vi "read_data.vi"(8 "error in (no error)":errorcluster, 11 "SGDClassifier in":refnum<class "SGDClassifier.lvclass">) -> (0 "error out":errorcluster, 2 "data":T1, 3 "SGDClassifier out":refnum<class "SGDClassifier.lvclass">)   [LabVIEW 2020, in "SGDClassifier.lvclass"]
uses:
  SGDClassifier.lvclass
  Controls/sgdclassifier_data.ctl
  SGDClassifier.lvclass/SGDClassifier.ctl
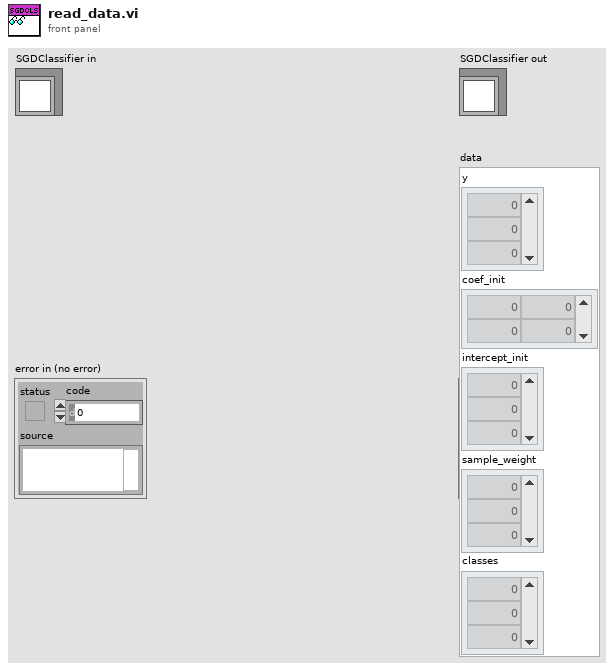
[diagram p1: front panel]
types:
  T1 = typedef "sgdclassifier_data.ctl" = cluster{"y":dbl[], "coef_init":dbl[][], "intercept_init":dbl[], "sample_weight":dbl[], "classes":dbl[]}
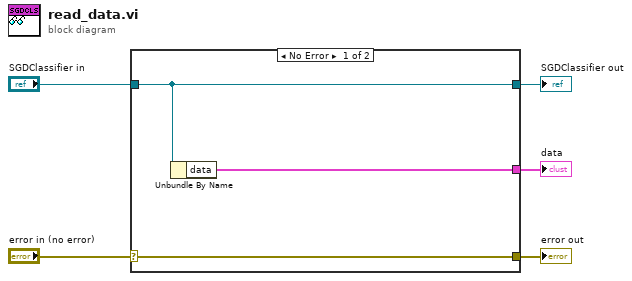
[diagram p0: block diagram]
diagram:
  n1 = case shown="No Error" "error in (no error)" {
    selector: "error in (no error)" -> [w8 w9]
    tunnel: [w8 w9] -> w4
    tunnel: [w7 w10] -> w2
    tunnel: "SGDClassifier in" -> [w7 w10]
    tunnel: [w6 _] -> w1
    frame No Error {
      n2 = Unbundle By Name(w7) -> ("data"=w6:T1)
    }
    frame Error {
    }
  }
  "error out" <- w4
  "SGDClassifier out" <- w2
  "data" <- w1
